vi "TestCollection.vi"() -> ()   [LabVIEW 2021, in "Collection.lvlib"]
uses:
  Collection.lvlib
  Class 1/Class 1.lvclass
  Class 2/Class 2.lvclass
  Class 1/SetNumeric.vi
  CollectionByValue/CollectionByValue.lvclass
panel:
  out "error out (no error)":errorcluster
  out "All Class 2":string[](array[string])
  out "error out (no error)":errorcluster
  out "All Class 1":string[](array[string])
  out "ClassName (Class 2)":string
  out "error out (error)":errorcluster
  out "ClassName (Class 1:2)":string
  out "found 2":bool
  out "ClassName (Class 2)":string
  out "found":bool
  out "ClassName (Class 1:1)":string
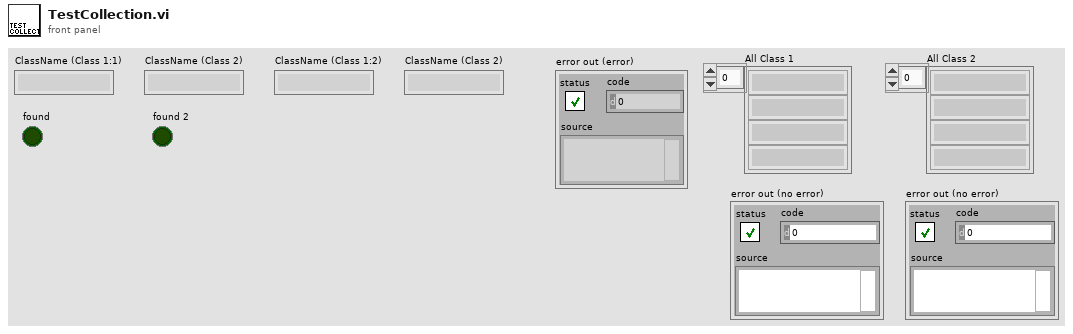
[diagram p1: front panel]
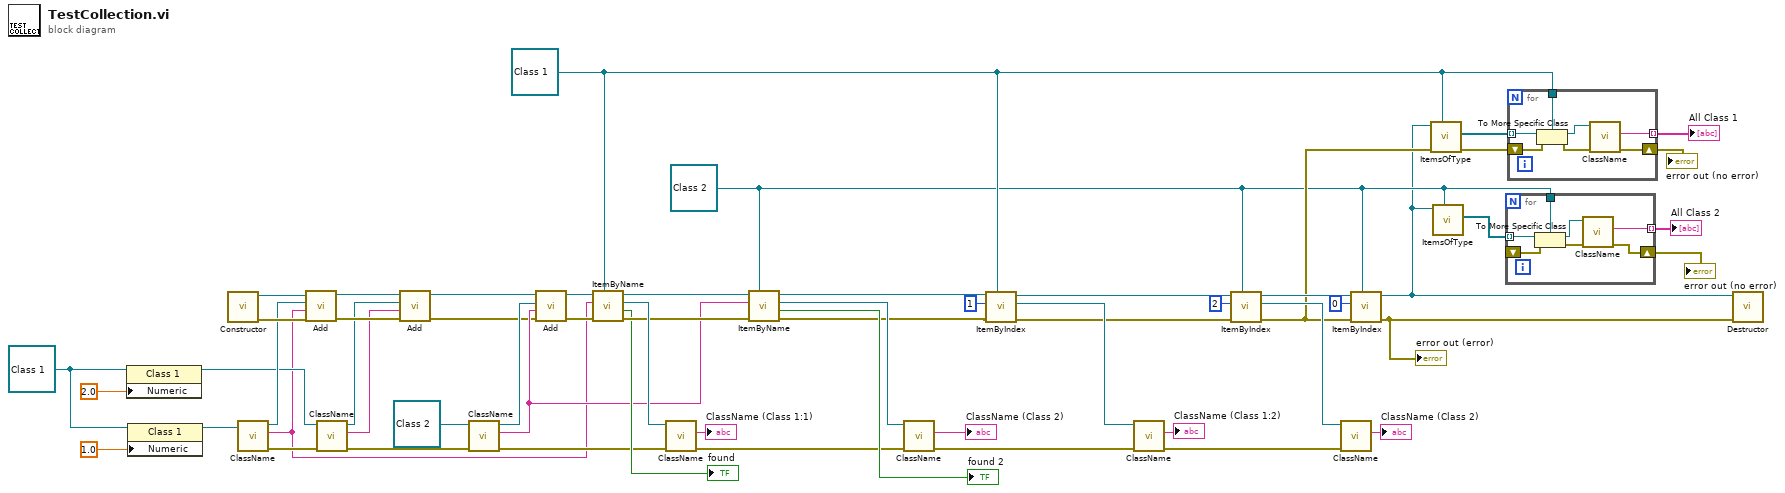
[diagram p0: block diagram]
diagram:
  w4 = refnum<class "Class 2.lvclass"> refnum ("Class 2.lvclass")
  w10 = refnum<class "Class 1.lvclass"> refnum ("Class 1.lvclass")
  w21 = refnum<class "Class 1.lvclass"> refnum ("Class 1.lvclass")
  n1 = property class="Class 1"(reference=w21, "Numeric"=2.0) -> (reference out=w20:refnum<class "Class 1.lvclass">)  [unwired: 1 in, 1 out]
  n2 = property class="Class 1"(reference=w21, "Numeric"=1.0) -> (reference out=w25:refnum<class "Class 1.lvclass">)  [unwired: 1 in, 1 out]
  n3 = call "Constructor.vi"() -> ("error out"=w57:errorcluster, "Collection out"=w58:refnum<class "CollectionByValue.lvclass">)  [unwired: 10 in]
  n4 = call-dynamic "ClassName.vi"("Class 1 in"=w25) -> ("error out"=w23:errorcluster, "ClassName"=w13:string, "Class 1 out"=w29:refnum<class "Class 1.lvclass">)  [unwired: 8 in]
  n5 = call "Add.vi"("error in (no error)"=w57, "Name"=w13, "LabVIEW Object"=w29, "Collection in"=w58) -> ("error out"=w19:errorcluster, "Collection out"=w17:refnum<class "CollectionByValue.lvclass">)  [unwired: 6 in]
  n6 = call-dynamic "ClassName.vi"("error in (no error)"=w23, "Class 1 in"=w20) -> ("error out"=w22:errorcluster, "ClassName"=w14:string, "Class 1 out"=w15:refnum<class "Class 1.lvclass">)  [unwired: 7 in]
  n7 = call "Add.vi"("error in (no error)"=w19, "Name"=w14, "LabVIEW Object"=w15, "Collection in"=w17) -> ("error out"=w18:errorcluster, "Collection out"=w16:refnum<class "CollectionByValue.lvclass">)  [unwired: 6 in]
  n8 = call-dynamic "ClassName.vi"("error in (no error)"=w22, "Class 2 in"=refnum<class "Class 2.lvclass"> refnum ("Class 2.lvclass")) -> ("error out"=w45:errorcluster, "ClassName"=w28:string, "Class 2 out"=w27:refnum<class "Class 2.lvclass">)  [unwired: 7 in]
  n9 = call "Add.vi"("error in (no error)"=w18, "Name"=w28, "LabVIEW Object"=w27, "Collection in"=w16) -> ("error out"=w54:errorcluster, "Collection out"=w55:refnum<class "CollectionByValue.lvclass">)  [unwired: 6 in]
  n10 = call "ItemByName.vi"("LabVIEW Object Type"=w10, "error in (no error)"=w54, "Name"=w13, "Collection in"=w55) -> ("error out"=w50:errorcluster, "found"=→"found":bool, "LabVIEW Object"=w53:refnum<class "Class 1.lvclass">, "Collection out"=w51:refnum<class "CollectionByValue.lvclass">)  [unwired: 4 in]
  n11 = call-dynamic "ClassName.vi"("error in (no error)"=w45, "Class 1 in"=w53) -> ("error out"=w44:errorcluster, "ClassName"=→"ClassName (Class 1:1)":string)  [unwired: 7 in, 1 out]
  n12 = call "ItemByName.vi"("LabVIEW Object Type"=w4, "error in (no error)"=w50, "Name"=w28, "Collection in"=w51) -> ("error out"=w43:errorcluster, "found"=→"found 2":bool, "LabVIEW Object"=w48:refnum<class "Class 2.lvclass">, "Collection out"=w42:refnum<class "CollectionByValue.lvclass">)  [unwired: 4 in]
  n13 = call-dynamic "ClassName.vi"("error in (no error)"=w44, "Class 2 in"=w48) -> ("error out"=w38:errorcluster, "ClassName"=→"ClassName (Class 2)":string)  [unwired: 7 in, 1 out]
  n14 = call "ItemByIndex.vi"("LabVIEW Object Type"=w10, "error in (no error)"=w43, "Index"=1, "Collection in"=w42) -> ("error out"=w37:errorcluster, "LabVIEW Object"=w40:refnum<class "Class 1.lvclass">, "Collection out"=w36:refnum<class "CollectionByValue.lvclass">)  [unwired: 4 in, 1 out]
  n15 = call-dynamic "ClassName.vi"("error in (no error)"=w38, "Class 1 in"=w40) -> ("error out"=w33:errorcluster, "ClassName"=→"ClassName (Class 1:2)":string)  [unwired: 7 in, 1 out]
  n16 = call "ItemByIndex.vi"("LabVIEW Object Type"=w4, "error in (no error)"=w37, "Index"=2, "Collection in"=w36) -> ("error out"=w8:errorcluster, "LabVIEW Object"=w34:refnum<class "Class 2.lvclass">, "Collection out"=w32:refnum<class "CollectionByValue.lvclass">)  [unwired: 4 in, 1 out]
  n17 = call-dynamic "ClassName.vi"("error in (no error)"=w33, "Class 2 in"=w34) -> ("ClassName"=→"ClassName (Class 2)":string)  [unwired: 7 in, 2 out]
  n18 = call "ItemByIndex.vi"("LabVIEW Object Type"=w4, "error in (no error)"=w8, "Index"=0, "Collection in"=w32) -> ("error out"=w26:errorcluster, "Collection out"=w1:refnum<class "CollectionByValue.lvclass">)  [unwired: 4 in, 2 out]
  "error out (error)" <- w26
  n19 = call "ItemsOfType.vi"("LabVIEW Object Type"=w10, "error in (no error)"=w8, "Collection in"=w1) -> ("error out"=w9:errorcluster, "LabVIEW Objects"=w11:refnum<class>[])  [unwired: 5 in, 2 out]
  n20 = call "ItemsOfType.vi"("LabVIEW Object Type"=w4, "Collection in"=w1) -> ("LabVIEW Objects"=w5:refnum<class>[])  [unwired: 6 in, 3 out]
  n21 = for {
    tunnel: w5 -> [w65] mode=indexing
    tunnel: w4 -> [w64]
    shift-right: [w61] -> w2
    shift-left: _ -> [w63]
    tunnel: [w59] -> w3 mode=indexing
    n22 = To More Specific Class(target class=w64, reference=w65, error in=w63) -> (specific class reference=w60:refnum<class "Class 2.lvclass">, error out=w62:errorcluster)
    n23 = call-dynamic "ClassName.vi"("error in (no error)"=w62, "Class 2 in"=w60) -> ("error out"=w61:errorcluster, "ClassName"=w59:string)  [unwired: 7 in, 1 out]
  }
  "All Class 2" <- w3
  "error out (no error)" <- w2
  n24 = for {
    tunnel: w11 -> [w72] mode=indexing
    tunnel: w10 -> [w71]
    shift-right: [w68] -> w6
    shift-left: w9 -> [w67]
    tunnel: [w66] -> w7 mode=indexing
    n25 = To More Specific Class(target class=w71, reference=w72, error in=w67) -> (specific class reference=w70:refnum<class "Class 1.lvclass">, error out=w69:errorcluster)
    n26 = call-dynamic "ClassName.vi"("error in (no error)"=w69, "Class 1 in"=w70) -> ("error out"=w68:errorcluster, "ClassName"=w66:string)  [unwired: 7 in, 1 out]
  }
  "All Class 1" <- w7
  "error out (no error)" <- w6
  n27 = call "Destructor.vi"("error in (no error)"=w26, "Collection in"=w1) -> ()  [unwired: 9 in, 1 out]
